vi "SerializeEmbeddedDataLines.vi"(11 "Embedded Data Lines":cluster{"mipiDataType":u8, "Line Data":u8[]}[](array[cluster])) -> (2 "length":i32, 3 "Serialized embedded data":string)   [LabVIEW 2021]
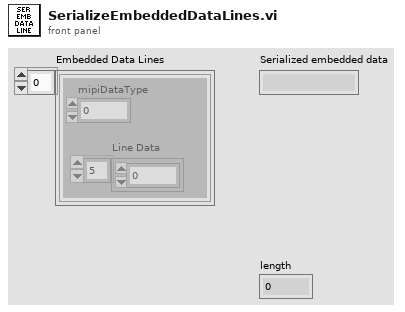
[diagram p1: front panel]
types:
  T1 = enum16{"big-endian, network order", "native, host order", "little-endian"}
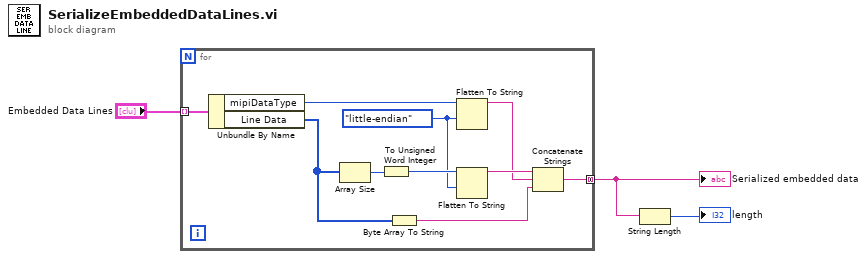
[diagram p0: block diagram]
diagram:
  n1 = for {
    tunnel: "Embedded Data Lines" -> [w13] mode=indexing
    tunnel: [w4] -> w2 mode=concatenating
    w9 = T1."little-endian" ("byte order (0:big-endian, network order)")
    n2 = Unbundle By Name(w13) -> ("mipiDataType"=w12:u8, "Line Data"=w8:u8[])
    n3 = Array Size(array=w8) -> (size(s)=w11:i32)
    n4 = To Unsigned Word Integer(number=w11) -> (unsigned 16bit integer=w10:u16)
    n5 = Byte Array To String(unsigned byte array=w8) -> (string=w5:string)
    n6 = Flatten To String(anything=w12, byte order (0:big-endian, network order)=w9) -> (data string=w6:string)  [unwired: 2 in, 2 out]
    n7 = Flatten To String(anything=w10, byte order (0:big-endian, network order)=w9) -> (data string=w7:string)  [unwired: 2 in, 2 out]
    n8 = Concatenate Strings(w7, w6, w5) -> (w4:string)
  }
  "Serialized embedded data" <- w2
  n9 = String Length(string=w2) -> (length=→"length":i32)
